vi "Strip Comments.vi"(8 "error in (no error)":errorcluster, 11 "String":string) -> (0 "error out":errorcluster, 1 "number of comments":i32, 3 "String out":string)   [LabVIEW 2015, in "YAML Parser.lvclass"]
uses:
  YAML Parser.lvclass
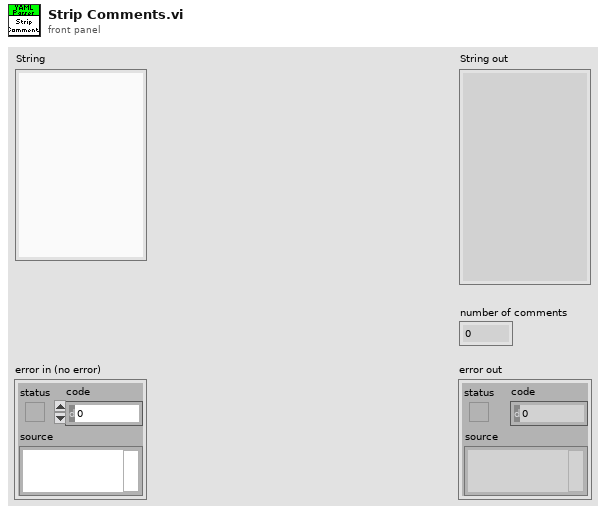
[diagram p1: front panel]
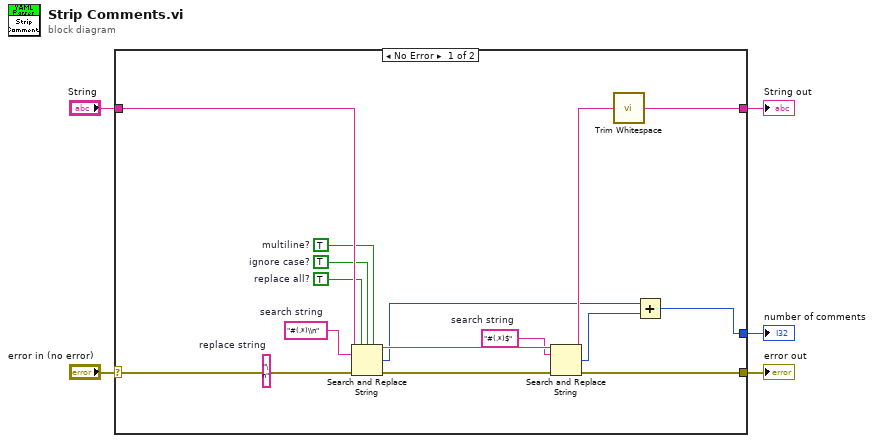
[diagram p0: block diagram]
diagram:
  n1 = case shown="No Error" "error in (no error)" {
    selector: "error in (no error)" -> [w21 w23]
    tunnel: [w12 w23] -> w4
    tunnel: [w6 w22] -> w2
    tunnel: "String" -> [w20 w22]
    tunnel: [w7 _] -> w1
    frame No Error {
      w10 = "#(.*)$"  # search string
      w14 = "\n"  # replace string
      w15 = "#(.*)\\n"  # search string
      w16 = TRUE  # multiline?
      w17 = TRUE  # ignore case?
      w18 = TRUE  # replace all?
      n2 = Search and Replace String(replace all?=w18, case sensitive?=w17, multiline?=w16, input string=w20, search string=w15, replace string=w14, error in=w21) -> (result string=w19:string, number of replacements=w8:i32, error out=w13:errorcluster)  [unwired: 1 in, 1 out]
      n3 = Search and Replace String(input string=w19, search string=w10, error in=w13) -> (result string=w11:string, number of replacements=w9:i32, error out=w12:errorcluster)  [unwired: 5 in, 1 out]
      n4 = call <vilib>:"Trim Whitespace.vi"("string"=w11) -> ("trimmed string"=w6:string)  [unwired: 1 in]
      n5 = Add(x=w8, y=w9) -> (x+y=w7:i32)
    }
    frame Error {
    }
  }
  "error out" <- w4
  "String out" <- w2
  "number of comments" <- w1
